vi "custom_painter.vi"(1 "Point":cluster{"X":i32, "Y":i32}, 2 "Color":u32(colorbox)=6618880, 3 "Picture in":picture) -> (0 "Picture out":picture)   [LabVIEW 2017]
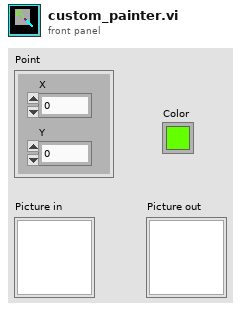
[diagram p1: front panel]
types:
  T1 = cluster{"Width":u16, "Style":enum32{"Solid", "Dash", "Dot", "DashDot", "DashDotDot"}}
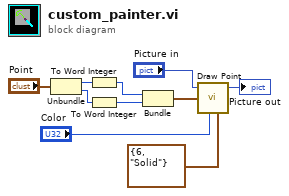
[diagram p0: block diagram]
diagram:
  n1 = Unbundle("Point") -> ("X"=w9:i32, "Y"=w8:i32)
  n2 = To Word Integer(number=w9) -> (16bit integer=w7:i16)
  n3 = To Word Integer(number=w8) -> (16bit integer=w6:i16)
  n4 = Bundle(w7, w6) -> (w5:cluster{i16, i16})  [unwired: 1 in]
  n5 = call <vilib>:"Draw Point.vi"("picture"="Picture in", "point(x,y)"=w5, "color(black)"="Color", "pen"=T1 {"Width"=6, "Style"=enum."Solid"}) -> ("new picture"=→"Picture out":picture)  [unwired: 5 in]
